vi "Matches serialisation type.vi"(8 "error in (no error)":errorcluster, 10 "Serialisation":T1, 11 "WAMP Client in":refnum<class "WAMP Client.lvclass">) -> (0 "error out":errorcluster, 2 "Matches?":bool, 3 "WAMP Client out":refnum<class "WAMP Client.lvclass">)   [LabVIEW 2020, in "wamplv.lvlib" / "WAMP Client.lvclass"]
uses:
  WAMP Client.lvclass
  WAMP Client.lvclass/WAMP Client.ctl
  <vilib>/ErrorRing/Error Ring.xnode
  <vilib>/Utility/error.llb/Error Cluster From Error Code.vi
  API/TypeDefs/Serialisation.ctl
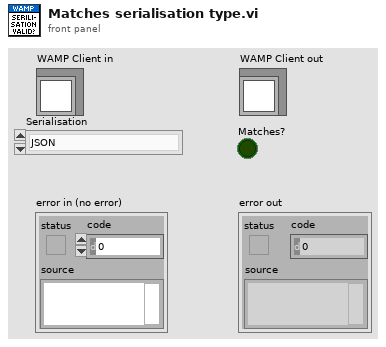
[diagram p1: front panel]
types:
  T1 = typedef "wamplv.lvlib/WAMP Client.lvclass/Serialisation.ctl" = enum16{"JSON", "MessagePack"}
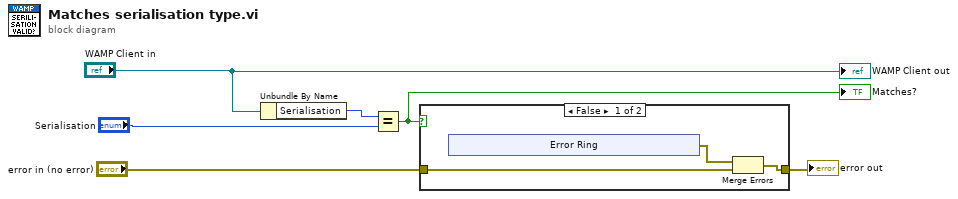
[diagram p0: block diagram]
diagram:
  n1 = Unbundle By Name("WAMP Client in") -> ("Serialisation"=w6:T1)
  n2 = Equal?(x=w6, y="Serialisation") -> (x = y?=w1:bool)
  "Matches?" <- w1
  n3 = case shown="False" w1 {
    tunnel: "error in (no error)" -> [w8 w14]
    tunnel: [w9 w14] -> w3
    frame False {
      n4 = xnode "Error Ring"() -> ("error out"=w7:errorcluster)
      n5 = Merge Errors(w7, w8) -> (w9:errorcluster)
    }
    frame True {
    }
  }
  "error out" <- w3
  "WAMP Client out" <- "WAMP Client in"
